vi "MListbox Align Column.vi"(6 "Active Cell:Cell Justification":enum16{"Left", "Center", "Right"}(ring), 8 "error in (no error)":errorcluster, 10 "Column Index":i16=-1, 11 "Multicolumn ListBox in":refnum<class "Multicolumn ListBox.lvclass">) -> (0 "error out":errorcluster, 3 "Multicolumn ListBox out":refnum<class "Multicolumn ListBox.lvclass">)   [LabVIEW 2018, in "Multicolumn ListBox.lvclass"]
uses:
  Multicolumn ListBox.lvclass
  Multicolumn ListBox.lvclass/Multicolumn ListBox.ctl
  <vilib>/Utility/miscctls.llb/LVRowAndColumnTypeDef.ctl
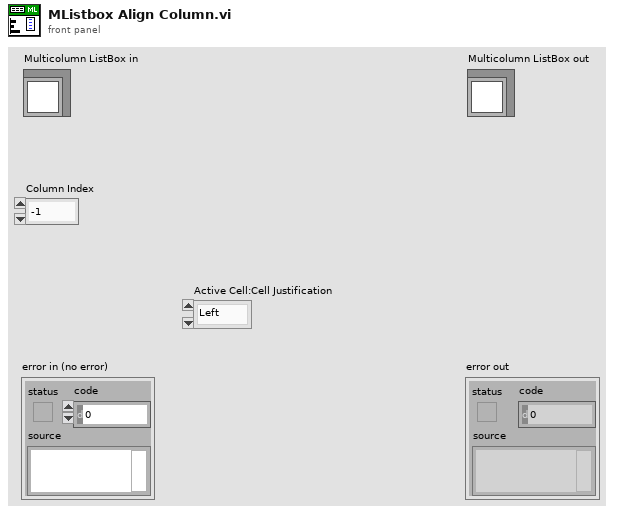
[diagram p1: front panel]
types:
  T1 = typedef "LVRowAndColumnTypeDef.ctl" = cluster{"Row":i32, "Column":i32}
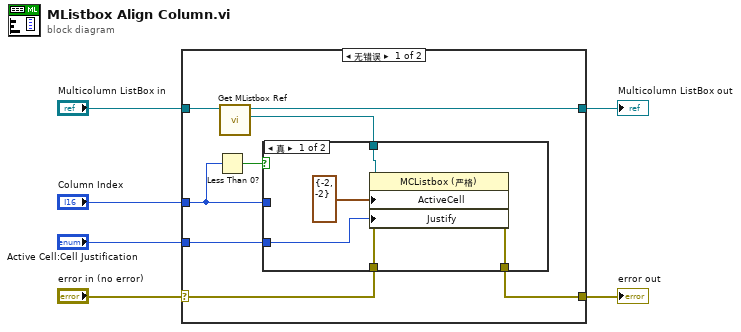
[diagram p0: block diagram]
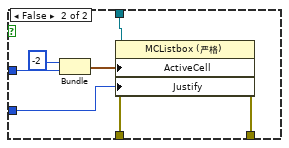
[diagram p2: hidden frame]
diagram:
  n1 = case shown="无错误" "error in (no error)" {
    selector: "error in (no error)" -> [w9 w28]
    tunnel: [w8 w28] -> w5
    tunnel: [w13 w27] -> w3
    tunnel: "Multicolumn ListBox in" -> [w14 w27]
    tunnel: "Column Index" -> [w7 _]
    tunnel: "Active Cell:Cell Justification" -> [w11 _]
    frame No Error {
      n2 = Less Than 0?(x=w7) -> (x < 0?=w10:bool)
      n3 = call "Get MListbox Ref.vi"("Multicolumn ListBox in"=w14) -> ("MListbox Ref"=w12:refnum<vi>, "Multicolumn ListBox out"=w13:refnum<class "Multicolumn ListBox.lvclass">)  [unwired: 8 in, 1 out]
      n4 = case shown="真" w10 {
        tunnel: w12 -> [w19 w26]
        tunnel: w11 -> [w17 w25]
        tunnel: w9 -> [w16 w24]
        tunnel: [w15 w23] -> w8
        tunnel: w7 -> [_ w22]
        frame True {
          n5 = property class="MCListbox (严格)"(reference=w19, error in=w16, "ActiveCell"=T1 {"Row"=-2, "Column"=-2} ("Active Cell:Active Cell"), "Justify"=w17) -> (error out=w15:errorcluster)  [unwired: 1 out]
        }
        frame False {
          n6 = Bundle(-2, "Column Index"=w22) -> (w21:cluster{i32, "Column Index":i16})  [unwired: 1 in]
          n7 = property class="MCListbox (严格)"(reference=w26, error in=w24, "ActiveCell"=w21, "Justify"=w25) -> (error out=w23:errorcluster)  [unwired: 1 out]
        }
      }
    }
    frame Error {
    }
  }
  "error out" <- w5
  "Multicolumn ListBox out" <- w3
